vi "set_voltages.vi"(4 "Vy min(V)":dbl, 6 "Vy max(V)":dbl, 8 "error in (no error)":errorcluster, 9 "Vz min(V)":dbl, 10 "Vz max(V)":dbl, 11 "TrajectoryAK101022Resonance in":refnum<class "TrajectoryAK101022Resonance.lvclass">) -> (0 "error out":errorcluster, 3 "TrajectoryAK101022Resonance out":refnum<class "TrajectoryAK101022Resonance.lvclass">)   [LabVIEW 2010, in "TrajectoryAK101022Resonance.lvclass"]
uses:
  TrajectoryAK101022Resonance.lvclass
  TrajectoryAK101022Resonance.lvclass/TrajectoryAK101022Resonance.ctl
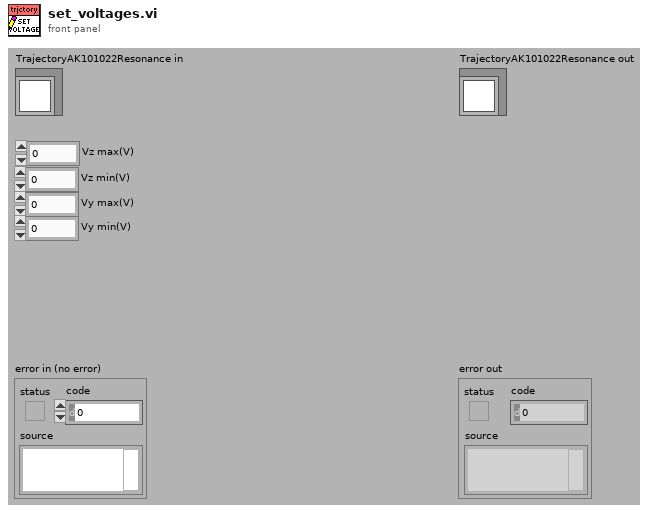
[diagram p1: front panel]
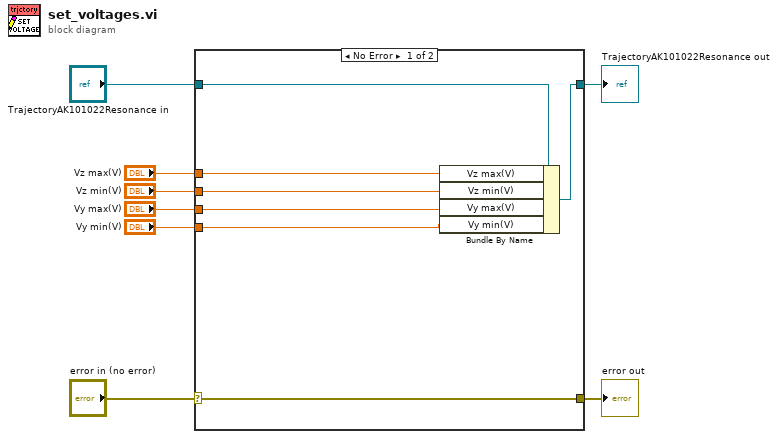
[diagram p0: block diagram]
diagram:
  n1 = case shown="No Error" "error in (no error)" {
    selector: "error in (no error)" -> [w15 w16]
    tunnel: [w15 w16] -> w7
    tunnel: [w13 w17] -> w5
    tunnel: "TrajectoryAK101022Resonance in" -> [w14 w17]
    tunnel: "Vz max(V)" -> [w9 _]
    tunnel: "Vz min(V)" -> [w12 _]
    tunnel: "Vy max(V)" -> [w11 _]
    tunnel: "Vy min(V)" -> [w10 _]
    frame No Error {
      n2 = Bundle By Name(cluster=w14, "Vz max(V)"=w9, "Vz min(V)"=w12, "Vy max(V)"=w11, "Vy min(V)"=w10) -> (w13:refnum<class "TrajectoryAK101022Resonance.lvclass">)
    }
    frame Error {
    }
  }
  "error out" <- w7
  "TrajectoryAK101022Resonance out" <- w5
